vi "Opponent.vi"(11 "Element in":refnum<class "Arilou.lvclass">) -> (2 "Player Type":T1, 3 "Opponent out":refnum<class "Element.lvclass">)   [LabVIEW 2021, in "Ship.lvclass"]
uses:
  Ship.lvclass
  Ships/Arilou/Arilou.lvclass
  C:/dev/LabVIEW/LabMelee/Source/Application Specific/Element/Element.lvclass
  Element/Element.lvclass
  Element/Element.lvclass/Element.ctl
  Ship.lvclass/Ship.ctl
  C:/dev/LabVIEW/LabMelee/Source/Application Specific/Ship/Ship.lvclass
  C:/dev/LabVIEW/LabMelee/Source/Application Specific/Ships/Arilou/Arilou.lvclass
  Globals.vi
  Element/Player Type.ctl
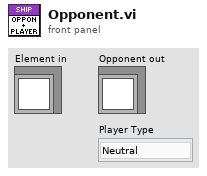
[diagram p1: front panel]
types:
  T1 = typedef "Element.lvclass/Player Type.ctl" = enum16{"Neutral", "Player 1", "Player 2"}
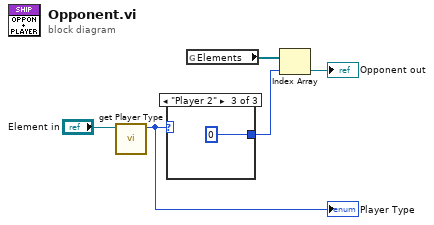
[diagram p0: block diagram]
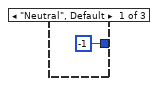
[diagram p2: hidden frame]
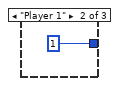
[diagram p3: hidden frame]
diagram:
  n1 = call "get Player Type.vi"("Element in"="Element in") -> ("Player Type"=w1:T1)  [unwired: 10 in]
  "Player Type" <- w1
  n2 = case shown="\"Player 2\"" w1 {
    tunnel: [-1 1 0] -> w3
    frame "Neutral", Default {
    }
    frame "Player 1" {
    }
    frame "Player 2" {
    }
  }
  n3 = global read "Globals.vi" "Elements"() -> (w2:refnum<class "Element.lvclass">[])
  n4 = Index Array(array=w2, index=w3) -> (element=→"Opponent out":refnum<class "Element.lvclass">)
